vi "Decode packed uint32.vi"(10 "Wire Type":T1, 11 "Data":u8[](array[numeric]) format="%.0x") -> (2 "error out":errorcluster, 3 "uint32":u32[](array[numeric]))   [LabVIEW 2020, in "LV-Proto.lvlib"]
uses:
  LV-Proto.lvlib
  Wire Type.ctl
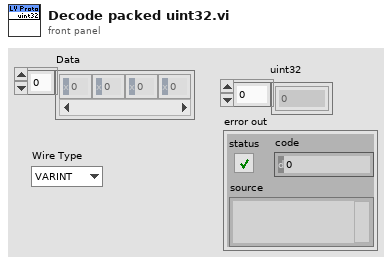
[diagram p1: front panel]
types:
  T1 = typedef "LV-Proto.lvlib/Wire Type.ctl" = enum8{"VARINT", "I64", "LEN", "SGROUP (Deprecated)", "EGROUP (Deprecated)", "I32"}
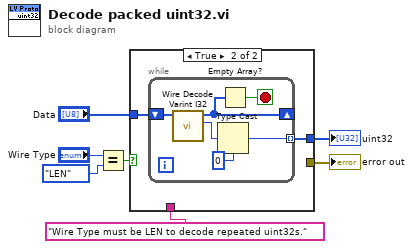
[diagram p0: block diagram]
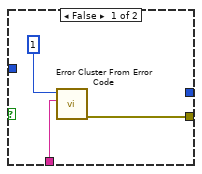
[diagram p2: hidden frame]
diagram:
  n1 = Equal?(x="Wire Type", y=Wire_Type."LEN") -> (x = y?=w3:bool)
  n2 = case shown="True" w3 {
    tunnel: [_ w11] -> w7
    tunnel: "Data" -> [_ w12]
    tunnel: [w9 _] -> w2
    tunnel: "Wire Type must be LEN to decode repeated uint32s." -> [w8 _]
    frame False {
      n3 = call <vilib>:"Error Cluster From Error Code.vi"("error message (\"\")"=w8, "error code (0)"=1) -> ("error out"=w9:errorcluster)  [unwired: 7 in]
    }
    frame True {
      n4 = while {
        tunnel: [w15] -> w11 mode=indexing
        shift-right: [w14] -> _
        shift-left: w12 -> [w18]
        stop <- w13 stop-if-true
        n5 = call "Wire Decode Varint I32.vi"("Buffer in"=w18) -> ("I32"=w17:i32, "Buffer"=w14:u8[])  [unwired: 9 in]
        n6 = Type Cast(type=u32 0, x=w17) -> (*(type *) &x=w15:u32)
        n7 = Empty Array?(array=w14) -> (empty?=w13:bool)
      }
    }
  }
  "uint32" <- w7
  "error out" <- w2
